vi "AlliGator FMB Get First Event.vi"(5 "Named Q Elements":T2[](array[typedef])) -> (0 "Data":variant, 1 "Named Q Event":T1=enum."Run Simulation", 2 "Named Q Elements":T2[](array[typedef]))   [LabVIEW 2021, in "AlliGator Fit Method Benchmark.lvlib"]
uses:
  AlliGator Fit Method Benchmark.lvlib
  AlliGator FMB Q Element.ctl
  AlliGator FMB Q Event List.ctl
  AlliGator FMB Global.vi
panel:
  # "see the License on the block diagram (Ctrl+E or Window:Show Block Diagram)"
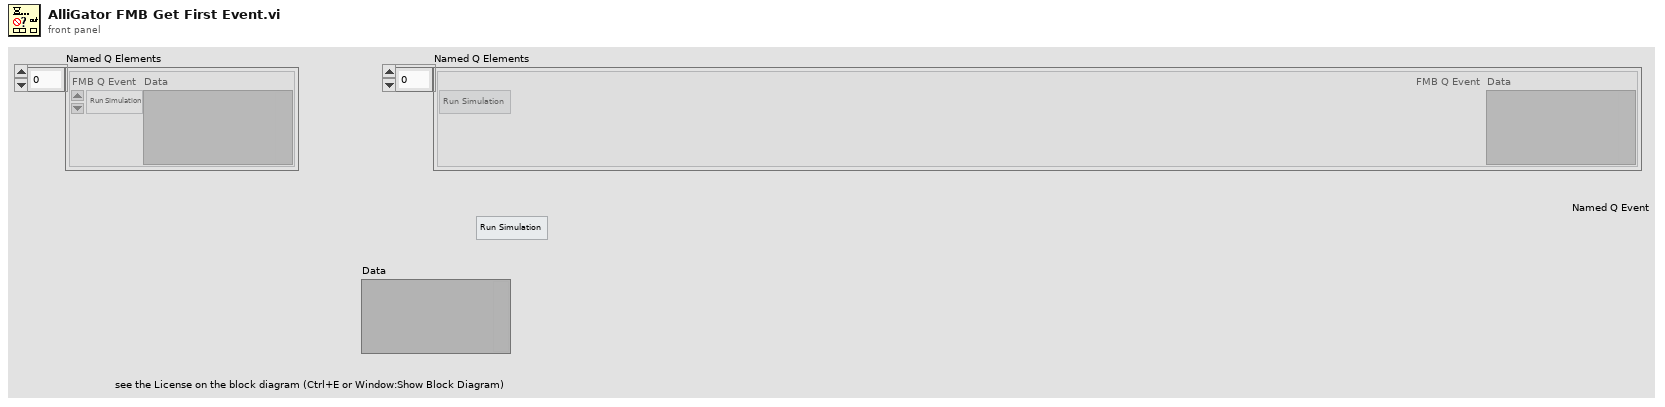
[diagram p1: front panel]
types:
  T1 = typedef "AlliGator Fit Method Benchmark.lvlib/AlliGator FMB Q Event List.ctl" = enum16{"Idle", "Initialization", "Update Script Simulation Parameters", "Single Simulation Prelude", "Run Simulation", "Update Histograms", "Update Script Simulation Output", "Graph Event", "Show Selected Decay", "Export Results", "Update # Processors Used", "Check Baseline", "Run Script", "End Script", "Init", "Abort", "Quit"}
  T2 = typedef "AlliGator Fit Method Benchmark.lvlib/AlliGator FMB Q Element.ctl" = cluster{"FMB Q Event":T1, "Data":variant}
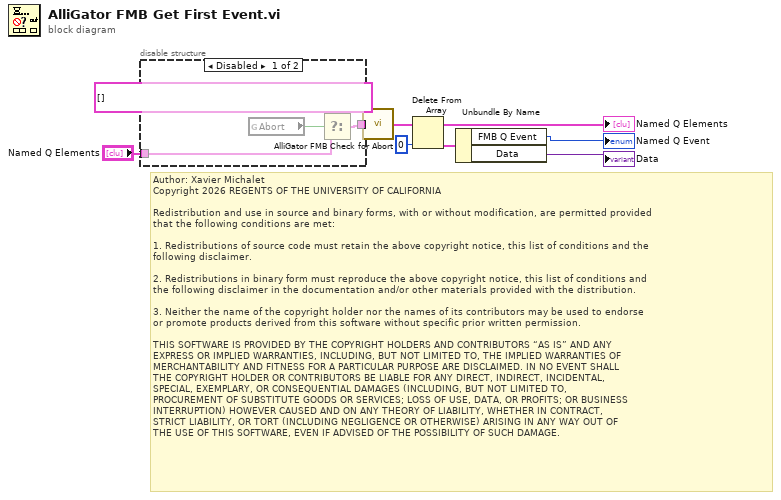
[diagram p0: block diagram]
diagram:
  # "Author: Xavier Michalet\nCopyright 2026 REGENTS OF THE UNIVERSITY OF CALIFORNIA\n\nRedistribution and use in source and binary forms, with or without modification, are permitted provided\nthat the following conditions are met:\n\n1. Redistributions of source code must retain the above copyright notice, this list of conditions and the\nfollowing disclaimer.\n\n2. Redistributions in binary form must reproduce the above copyright notice, this list of conditions and\nthe following disclaimer in the documentation and/or other materials provided with the distribution.\n\n3. Neither the name of the copyright holder nor the names of its contributors may be used to endorse \nor promote products derived from this software without specific prior written permission.\n\nTHIS SOFTWARE IS PROVIDED BY THE COPYRIGHT HOLDERS AND CONTRIBUTORS “AS IS” AND ANY \nEXPRESS OR IMPLIED WARRANTIES, INCLUDING, BUT NOT LIMITED TO, THE IMPLIED WARRANTIES OF\nMERCHANTABILITY AND FITNESS FOR A PARTICULAR PURPOSE ARE DISCLAIMED. IN NO EVENT SHALL\nTHE COPYRIGHT HOLDER OR CONTRIBUTORS BE LIABLE FOR ANY DIRECT, INDIRECT, INCIDENTAL, \nSPECIAL, EXEMPLARY, OR CONSEQUENTIAL DAMAGES (INCLUDING, BUT NOT LIMITED TO, \nPROCUREMENT OF SUBSTITUTE GOODS OR SERVICES; LOSS OF USE, DATA, OR PROFITS; OR BUSINESS\nINTERRUPTION) HOWEVER CAUSED AND ON ANY THEORY OF LIABILITY, WHETHER IN CONTRACT, \nSTRICT LIABILITY, OR TORT (INCLUDING NEGLIGENCE OR OTHERWISE) ARISING IN ANY WAY OUT OF\nTHE USE OF THIS SOFTWARE, EVEN IF ADVISED OF THE POSSIBILITY OF SUCH DAMAGE."
  n1 = disable-structure shown="Disabled" {
    disable-tunnel: [w11 w13] -> w7
    disable-tunnel: "Named Q Elements" -> [w10 w13]
    frame Disabled {
      n2 = global read "AlliGator FMB Global.vi" "Abort"() -> (w9:bool)
      n3 = Select(t=T2[] [] ("array w/ subset deleted"), s=w9, f=w10) -> (s? t:f=w11:T2[])
    }
    frame Enabled {
    }
  }
  n4 = call "AlliGator FMB Check for Abort.vi"("Named Q Elements"=w7) -> ("Named Q Elements"=w8:T2[])
  n5 = Delete From Array(array=w8, index=0) -> (deleted portion=w5:T2, array with subset deleted=→"Named Q Elements":T2[])  [unwired: 1 in]
  n6 = Unbundle By Name(w5) -> ("FMB Q Event"=→"Named Q Event":T1, "Data"=→"Data":variant)
